vi "Data Logging Message Loop.vi"(8 "error in (no error)":errorcluster, 10 "Data Queue":refnum<queue>, 11 "Message Queues":T2) -> (0 "error out":errorcluster)   [LabVIEW 2026]
uses:
  support/Message Queue/All Message Queues.ctl
  support/Message Queue/Message Cluster.ctl
  controls/Waveforms.ctl
  support/Message Queue/Message Queue.lvlib
panel:
  out "data":T1
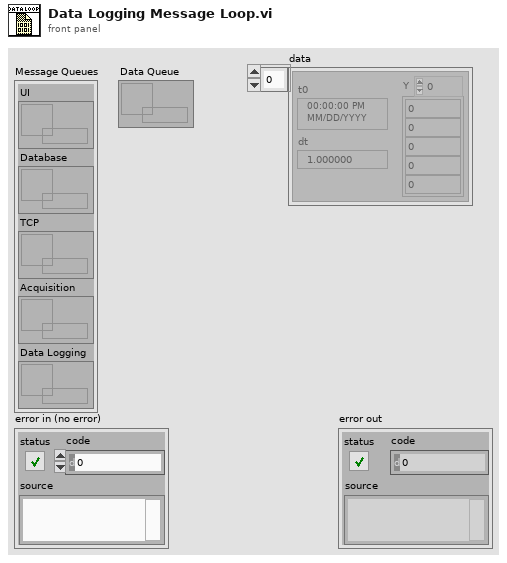
[diagram p1: front panel]
types:
  T1 = typedef "Waveforms.ctl" = waveform(dbl)[]
  T2 = typedef "Message Queue.lvlib/All Message Queues.ctl" = cluster{"UI":refnum<queue>, "Database":refnum<queue>, "TCP":refnum<queue>, "Acquisition":refnum<queue>, "Data Logging":refnum<queue>}
  T3 = enum16{"open", "open or create", "create or replace", "create", "open (read-only)"}
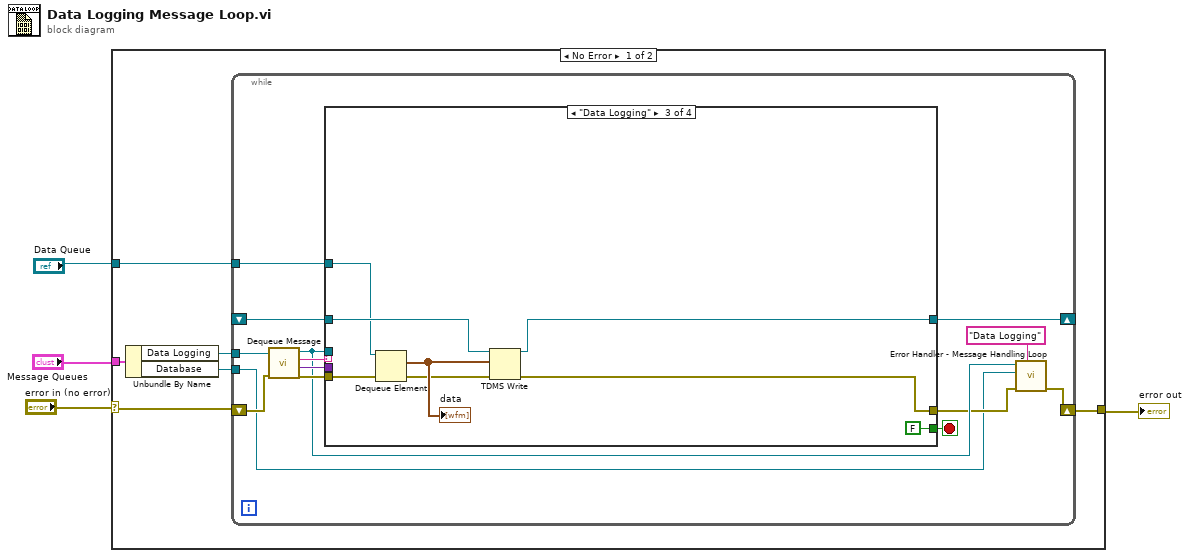
[diagram p0: block diagram]
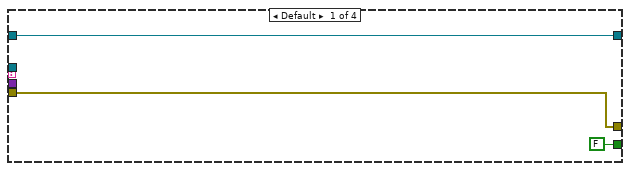
[diagram p2: hidden frame]
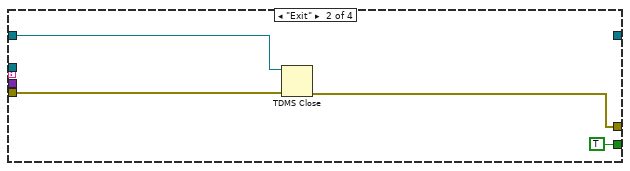
[diagram p3: hidden frame]
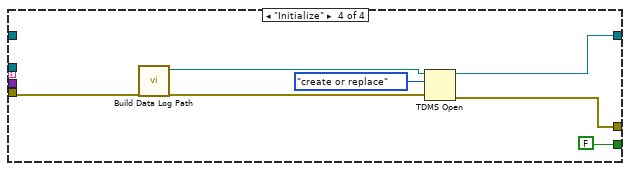
[diagram p4: hidden frame]
diagram:
  n1 = case shown="No Error" "error in (no error)" {
    selector: "error in (no error)" -> [w10 w47]
    tunnel: [w9 w47] -> w3
    tunnel: "Message Queues" -> [w8 _]
    tunnel: "Data Queue" -> [w6 _]
    frame No Error {
      n2 = Unbundle By Name(w8) -> ("Data Logging"=w7:refnum<queue>, "Database"=w5:refnum<queue>)
      n3 = while {
        shift-right: [w14] -> w9
        shift-left: w10 -> [w20]
        tunnel: w7 -> [w23]
        shift-right: [w22] -> _
        shift-left: _ -> [w21]
        tunnel: w6 -> [w13]
        tunnel: w5 -> [w12]
        stop <- w24 stop-if-true
        n4 = call "Dequeue Message.vi"("error in (no error)"=w20, "Message Queue"=w23) -> ("error out"=w19:errorcluster, "Message Data"=w17:variant, "Message"=w18:string, "dup Message Queue"=w16:refnum<queue>)  [unwired: 6 in]
        n5 = case shown="\"Data Logging\"" w18 {
          tunnel: w19 -> [w27 w30 w34 w42]
          tunnel: [w27 w29 w36 w40] -> w15
          tunnel: [FALSE TRUE FALSE FALSE] -> w24
          tunnel: [w25 _ w37 w43] -> w22
          tunnel: w21 -> [w25 w28 w38 _]
          tunnel: w17 -> [_ _ _ _]
          tunnel: w16 -> [_ _ _ _]
          tunnel: w13 -> [_ _ w35 _]
          frame Default {
          }
          frame "Exit" {
            n6 = TDMS Close(8:w30, 11:w28) -> (0:w29:errorcluster)  [unwired: 1 out]
          }
          frame "Data Logging" {
            n7 = Dequeue Element(queue=w35, error in (no error)=w34) -> (element=w33:waveform(dbl)[], error out=w32:errorcluster)  [unwired: 1 in, 2 out]
            "data" <- w33
            n8 = TDMS Write(0:w38, 9:w33, 11:w32) -> (4:w37:refnum<k34>, 15:w36:errorcluster)  [unwired: 3 in, 2 out]
          }
          frame "Initialize" {
            n9 = call "Build Data Log Path.vi"("error in (no error)"=w42) -> ("error out"=w41:errorcluster, "appended path"=w46:path)  [unwired: 9 in]
            n10 = TDMS Open(8:w41, 10:T3."create or replace" ("operation (0:open)"), 11:w46) -> (0:w40:errorcluster, 3:w43:refnum<k34>)  [unwired: 4 in]
          }
        }
        n11 = call "Error Handler - Message Handling Loop.vi"("Loop Name"="Data Logging", "error in (no error)"=w15, "Database"=w12, "Message Queue"=w16) -> ("dup error in"=w14:errorcluster)  [unwired: 6 in, 1 out]
      }
    }
    frame Error {
    }
  }
  "error out" <- w3
